vi "Lifter Hights.vi"() -> ()   [LabVIEW 2014]
panel:
  in  "Can Carry height":dbl=2800.0
  in  "Auton Set Point":dbl=2800.0
  in  "Can Height":dbl
  in  "Safe Drive  Height":dbl=573.0
  in  "HP Release Height":dbl=2300.0
  in  "HP Insert Height":dbl=3200.0
  in  "HP Indexer Collect":dbl=1050.0
  in  "2 tote release height 2":dbl=1500.0
  in  "1 tote release height":dbl=1300.0
  in  "END_HEIGHT":dbl=2500.0
  in  "set down tote":dbl=1500.0
  in  "top":dbl=3760.0
  in  "2 tote high":dbl
  in  "1 tote stack height":dbl=1488.0
  in  "FloorCollect":dbl
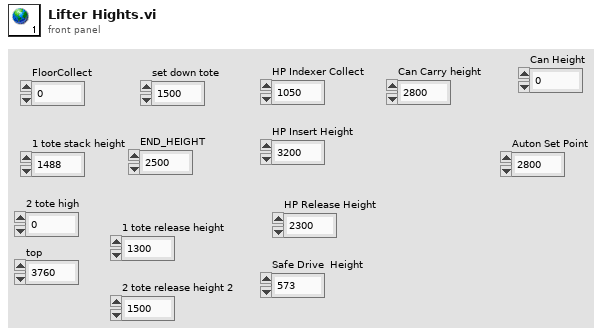
[diagram p1: front panel]
diagram:
